vi "Create Housekeeping Request.vi"(0 "Room Service Manager UI in":refnum<class "Room Service Manager UI.lvclass">, 11 "error in (no error)":errorcluster) -> (4 "Room Service Manager UI out":refnum<class "Room Service Manager UI.lvclass">, 15 "error out":errorcluster)   [LabVIEW 2023, in "Room Service Manager UI.lvlib" / "Room Service Manager UI.lvclass"]
uses:
  Room Service Manager UI.lvclass
  C:/Program Files/National Instruments/LabVIEW 2023/vi.lib/ActorFramework/Actor/Actor.lvclass
  <vilib>/ActorFramework/Actor/Actor.lvclass/Actor.ctl
  Room Service Manager UI.lvclass/Room Service Manager UI.ctl
  Room Service Types/Housekeeping/Housekeeping.lvclass
  C:/Users/bhaghyaraj/Trainings/NI Actor Framework/SDLC/Room Service Types/Room Service Base/Room Service Base.lvclass
  Central Data Manager/Central Data Manager/Room Service Type.ctl
  Room Service Manager UI Messages/Create Room Service Request Msg/Create Room Service Request Msg.lvclass/Create Room Service Request Msg.ctl
  <vilib>/ActorFramework/Message Enqueuer/Message Enqueuer.lvclass/Message Enqueuer.ctl
  <vilib>/ActorFramework/Message Enqueuer/Enqueue.vi
  Room Service Manager UI Messages/Create Room Service Request Msg/Create Room Service Request Msg.lvclass
  C:/Program Files/National Instruments/LabVIEW 2023/vi.lib/ActorFramework/Message/Message.lvclass
  <vilib>/ActorFramework/Message Priority Queue/Priority Enqueue.vi
  <vilib>/ActorFramework/Actor/Actor.lvclass
  Central Data Manager/Central Data Manager/Central Data Manager.lvclass
  C:/Users/bhaghyaraj/Trainings/NI Actor Framework/SDLC/UI Base/UI Base/UI Base.lvclass
  C:/Users/bhaghyaraj/Trainings/NI Actor Framework/SDLC/Room Service Manager UI/Room Service Manager UI/Room Service Manager UI.lvclass
  C:/Users/bhaghyaraj/Trainings/NI Actor Framework/SDLC/Room Service Types/Housekeeping/Housekeeping.lvclass
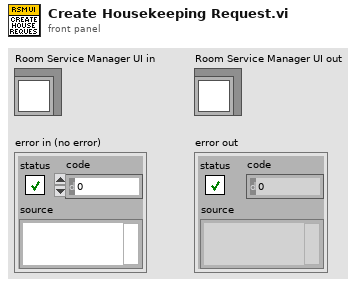
[diagram p1: front panel]
types:
  T1 = enum8{"Enabled", "Disabled", "Disabled and Grayed Out"}
  T2 = typedef "Central Data Manager.lvlib/Central Data Manager.lvclass/Room Service Type.ctl" = enum16{"Housekeeping", "Food Order", "Other Service"}
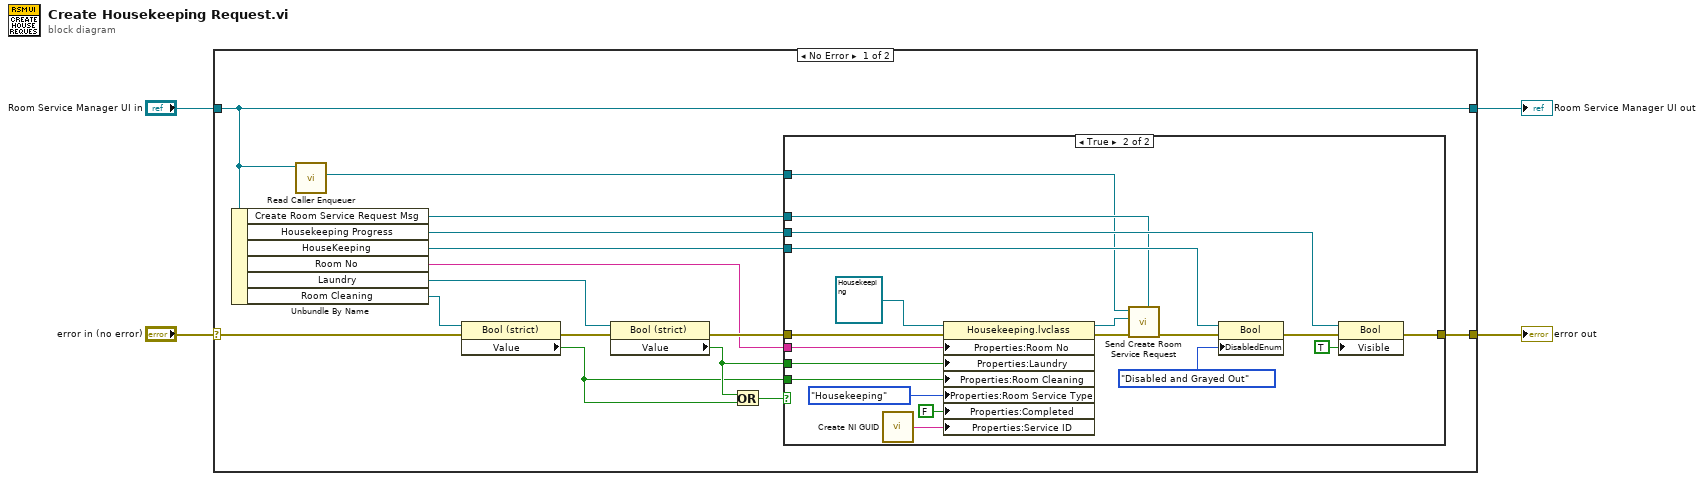
[diagram p0: block diagram]
diagram:
  n1 = case shown="No Error" "error in (no error)" {
    selector: "error in (no error)" -> [w19 w41]
    tunnel: [w13 w41] -> w3
    tunnel: [w14 w40] -> w1
    tunnel: "Room Service Manager UI in" -> [w14 w40]
    frame No Error {
      n2 = Unbundle By Name(w14) -> ("Create Room Service Request Msg"=w5:refnum<class "Create Room Service Request Msg.lvclass">, "Housekeeping Progress"=w6:refnum<vi>, "HouseKeeping"=w7:refnum<vi>, "Room No"=w12:string, "Laundry"=w16:refnum<vi>, "Room Cleaning"=w18:refnum<vi>)
      n3 = call <vilib>:"Read Caller Enqueuer.vi"("Actor"=w14) -> ("Caller Enqueuer"=w8:refnum<class "Message Enqueuer.lvclass">)  [unwired: 10 in]
      n4 = property class="Bool (strict)"(reference=w18, error in=w19) -> (error out=w17:errorcluster, "Value"=w10:bool)  [unwired: 1 out]
      n5 = property class="Bool (strict)"(reference=w16, error in=w17) -> (error out=w15:errorcluster, "Value"=w11:bool)  [unwired: 1 out]
      n6 = Or(x=w11, y=w10) -> (x .or. y?=w9:bool)
      n7 = case shown="True" w9 {
        tunnel: w15 -> [w20 w39]
        tunnel: [w20 w31] -> w13
        tunnel: w12 -> [_ w37]
        tunnel: w11 -> [_ w36]
        tunnel: w10 -> [_ w35]
        tunnel: w8 -> [_ w22]
        tunnel: w7 -> [_ w30]
        tunnel: w6 -> [_ w29]
        tunnel: w5 -> [_ w26]
        frame False {
        }
        frame True {
          n8 = call <vilib>:"Create NI GUID.vi"() -> ("NI GUID"=w21:string)
          n9 = property class="Housekeeping.lvclass"(reference=refnum<class "Housekeeping.lvclass"> refnum ("Room Service Types.lvlib:Housekeeping.lvclass"), error in=w39, "Properties:Room No"=w37, "Properties:Laundry"=w36, "Properties:Room Cleaning"=w35, "Properties:Room Service Type"=Room_Service_Type."Housekeeping" ("Room Service Type"), "Properties:Completed"=FALSE ("Completed"), "Properties:Service ID"=w21) -> (reference out=w23:refnum<class "Housekeeping.lvclass">, error out=w25:errorcluster)
          n10 = call "Send Create Room Service Request.vi"("Message Type"=w26, "error in (no error)"=w25, "Room Service"=w23, "Message Enqueuer"=w22) -> ("error out"=w24:errorcluster)  [unwired: 6 in, 1 out]
          n11 = property class="Bool"(reference=w30, error in=w24, "DisabledEnum"=T1."Disabled and Grayed Out" ("Disabled")) -> (error out=w32:errorcluster)  [unwired: 1 out]
          n12 = property class="Bool"(reference=w29, error in=w32, "Visible"=TRUE) -> (error out=w31:errorcluster)  [unwired: 1 out]
        }
      }
    }
    frame Error {
    }
  }
  "error out" <- w3
  "Room Service Manager UI out" <- w1
